vi "Main.vi"() -> ()   [LabVIEW 2020, in "Reentrancy.lvlib"]
uses:
  Reentrancy.lvlib
  Assignment backups/VISA/Typedefs/Data Cluster.ctl
  SubVI/clone.vi
panel:
  in  "Stop":bool
  out "Error out":errorcluster
  in  "Error in":errorcluster
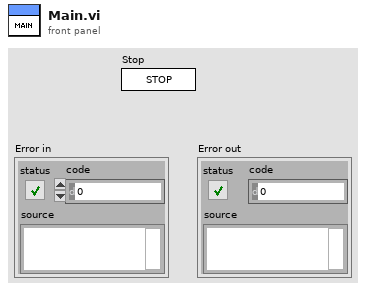
[diagram p1: front panel]
types:
  T1 = typedef "Data Cluster.ctl" = cluster{"Refrence Array":refnum<vi>[], "Clone no":i32}
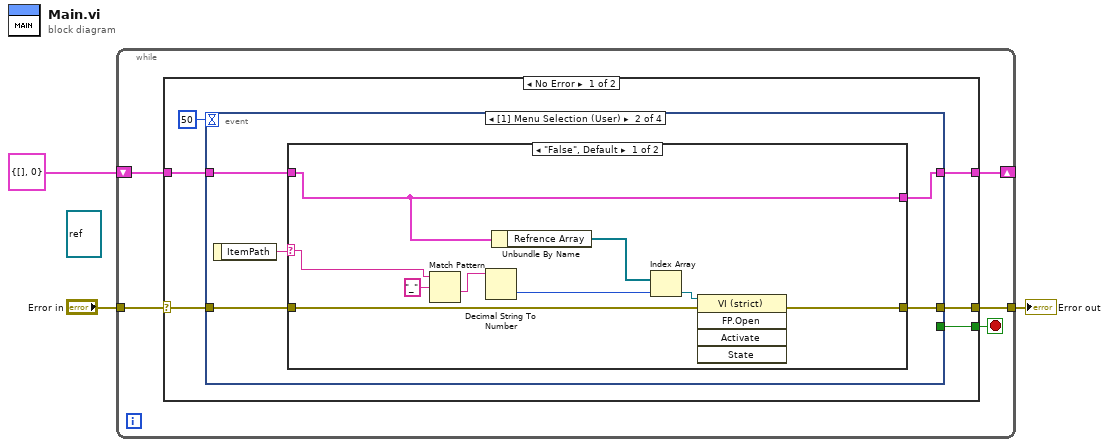
[diagram p0: block diagram]
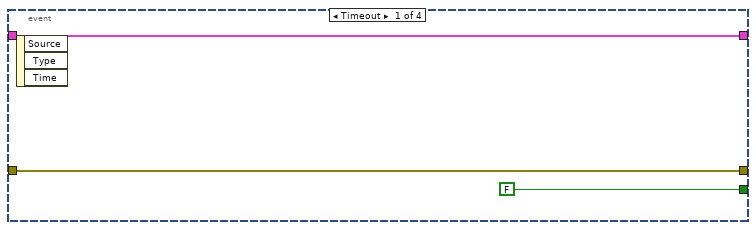
[diagram p2: hidden frame]
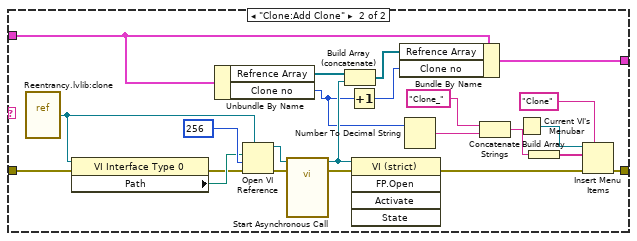
[diagram p3: hidden frame]
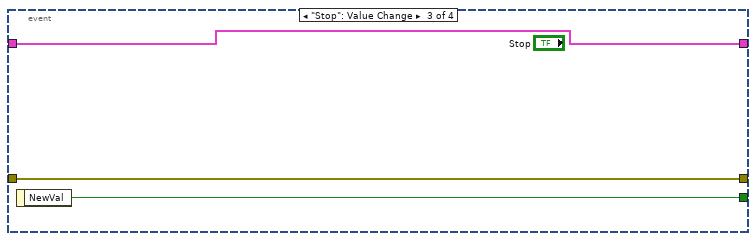
[diagram p4: hidden frame]
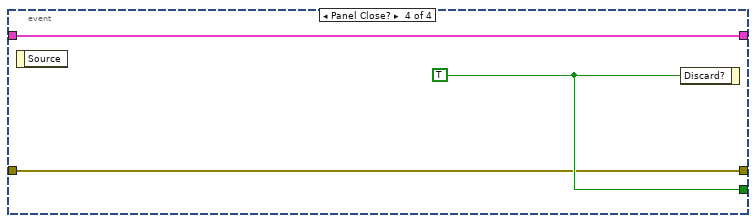
[diagram p5: hidden frame]
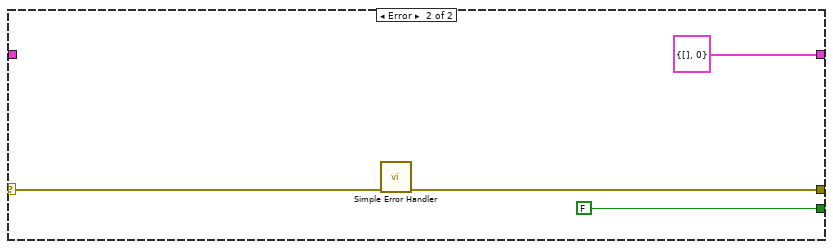
[diagram p6: hidden frame]
diagram:
  (unwired) refnum<vi> refnum ("reference out")
  n1 = while {
    tunnel: "Error in" -> [w8]
    tunnel: [w7] -> w2
    shift-right: [w4] -> _
    shift-left: T1 {"Refrence Array"=[], "Clone no"=0} -> [w5]
    stop <- w6 stop-if-true
    n2 = case shown="No Error" w8 {
      selector: w8 -> [w13 w64]
      tunnel: [w12 w63] -> w7
      tunnel: [w11 FALSE ("NewVal")] -> w6
      tunnel: w5 -> [w10 _]
      tunnel: [w9 T1 {"Refrence Array"=[], "Clone no"=0}] -> w4
      frame No Error {
        n3 = event shown="[1] Menu Selection (User)" {
          selector: _ -> [_ _ _ _]
          dyn-events: _ -> [_ _ _ _]
          timeout: 50 -> [_ _ _ _]
          tunnel: w13 -> [w17 w22 w57 w59]
          tunnel: [w17 w19 w57 w59] -> w12
          tunnel: [FALSE ("Discard?") _ w56 w60] -> w11
          tunnel: w10 -> [w15 w21 w55 w58]
          tunnel: [w15 w20 w55 w58] -> w9
          event Timeout {
            n4 = event-data() -> ()  [unwired: 1 in, 3 out]
          }
          event Menu Selection (User) {
            n5 = event-data() -> ("ItemPath"=w18:string)  [unwired: 1 in]
            n6 = case shown="\"False\", Default" w18 {
              selector: w18 -> [w25 _]
              tunnel: w22 -> [w26 w51]
              tunnel: w21 -> [w31 w41]
              tunnel: [w31 w40] -> w20
              tunnel: [w29 w32] -> w19
              frame "False", Default {
                n7 = Match Pattern(string=w25, regular expression="_") -> (after substring=w23:string)  [unwired: 1 in, 3 out]
                n8 = Decimal String To Number(string=w23) -> (number=w24:i32)  [unwired: 2 in, 1 out]
                n9 = Unbundle By Name(w31) -> ("Refrence Array"=w30:refnum<vi>[])
                n10 = Index Array(array=w30, index=w24) -> (element=w28:refnum<vi>)
                n11 = invoke class="VI (strict)" method="FP.Open"(reference=w28, error in=w26) -> (error out=w29:errorcluster)  [unwired: 3 in, 4 out]
              }
              frame "Clone:Add Clone" {
                n12 = vi-ref "Reentrancy.lvlib:clone.vi"() -> (w45:refnum<vi>)
                n13 = property class="VI Interface Type 0"(reference=w45, error in=w51) -> (error out=w49:errorcluster, "Path"=w50:path)  [unwired: 1 out]
                n14 = Unbundle By Name(w41) -> ("Refrence Array"=w43:refnum<vi>[], "Clone no"=w38:i32)
                n15 = Open VI Reference(type specifier VI Refnum (for type only)=w45, vi path=w50, options=256, error in (no error)=w49) -> (vi reference=w54:refnum<vi>, error out=w53:errorcluster)  [unwired: 2 in]
                n16 = call-by-ref "Start Asynchronous Call"(reference=w54, error in=w53) -> (reference out=w44:refnum<vi>, error out=w46:errorcluster)  [unwired: 12 in, 4 out]
                n17 = Build Array (concatenate)(w43, w44) -> (w42:refnum<vi>[])
                n18 = Increment(x=w38) -> (x+1=w39:i32)
                n19 = invoke class="VI (strict)" method="FP.Open"(reference=w44, error in=w46) -> (error out=w34:errorcluster)  [unwired: 3 in, 4 out]
                n20 = Bundle By Name(cluster=w41, "Refrence Array"=w42, "Clone no"=w39) -> (w40:T1)
                n21 = Number To Decimal String(number=w38) -> (decimal integer string=w36:string)  [unwired: 1 in]
                n22 = Concatenate Strings("Clone_", w36) -> (w35:string)
                n23 = Current VI's Menubar() -> (w48:refnum<k9>)
                n24 = Build Array(w35) -> (w33:string[])
                n25 = Insert Menu Items(5:"Clone" ("menu tag"), 6:w34, 8:w33, 9:w48) -> (0:w32:errorcluster)  [unwired: 2 in, 2 out]
              }
            }
          }
          event "Stop": Value Change {
            n26 = event-data() -> ("NewVal"=w56:bool)  [unwired: 1 in]
          }
          event Panel Close? {
            w60 = TRUE ("Discard?")
            n27 = event-data() -> ()  [unwired: 1 in, 1 out]
            n28 = event-data("Discard?"=w60) -> ()  [unwired: 1 in, 1 out]
          }
        }
      }
      frame Error {
        n29 = call <vilib>:"Simple Error Handler.vi"("error in (no error)"=w64) -> ("error out"=w63:errorcluster)  [unwired: 4 in, 4 out]
      }
    }
  }
  "Error out" <- w2
